vi "PhotonTrackedTarget_Newt.vi"(0 "Pitch":dbl, 1 "Yaw":dbl, 5 "Area":dbl, 7 "Skew":dbl, 9 "FiducalId":i32, 11 "CameraToTarget":T2={"TRANSLATION"={"X"=0.0, "Y"=0.0}, "ROTATION"={"VALUE"=0.0, "COS"=1.0, "SIN"=0.0}, "xF"=FALSE} {"ROTATION"."SIN" format="%13.4f"; "ROTATION"."COS" format="%13.4f"; "ROTATION"."VALUE" format="%13.4f"; "TRANSLATION"."Y" format="%14.3f"; "TRANSLATION"."X" format="%14.3f"}, 13 "TargetCorners":T1[](array[typedef])) -> (4 "TrackedTarget":T5={"Yaw"=0.0, "Pitch"=0.0, "Area"=0.0, "Skew"=0.0, "TargetCorners"=[], "CameraToTarget"={"TRANSLATION"={"X"=0.0, "Y"=0.0}, "ROTATION"={"VALUE"=0.0, "COS"=1.0, "SIN"=0.0}, "xF"=FALSE}, "FiducialId"=0} {"CameraToTarget"."ROTATION"."SIN" format="%13.4f"; "CameraToTarget"."ROTATION"."COS" format="%13.4f"; "CameraToTarget"."ROTATION"."VALUE" format="%13.4f"; "CameraToTarget"."TRANSLATION"."Y" format="%14.3f"; "CameraToTarget"."TRANSLATION"."X" format="%14.3f"})   [LabVIEW 2020, in "PhotonVisionLib.lvlib"]
doc: "Create a new TracedTarget data cluster\n\nInputs:\n - Yaw -- \n - Pitch -- \n - Area -- \n - Skew -- \n - CameraToTarget -- Transform2d\n - TargetCorners -- Array of 4 corners.\n\nOutputs:\n - TrackedTarget -- Created TrackedTarget cluster."
uses:
  PhotonVisionLib.lvlib
  TypeDef/PhotonTrackedTargetType.ctl
  TypeDef/TargetCornerType.ctl
  <vilib>/Rock Robotics/WPI/ThirdParty/JAS_Junk/TrajLib/TypeDef/TRANSFORM2D.ctl
  <vilib>/Rock Robotics/WPI/ThirdParty/JAS_Junk/TrajLib/TypeDef/TRANSLATION2D.ctl
  <vilib>/Rock Robotics/WPI/ThirdParty/JAS_Junk/TrajLib/TypeDef/ROTATION2D.ctl
  <vilib>/Rock Robotics/WPI/ThirdParty/JAS_Junk/TrajLib/Trajectory_Library.lvlib
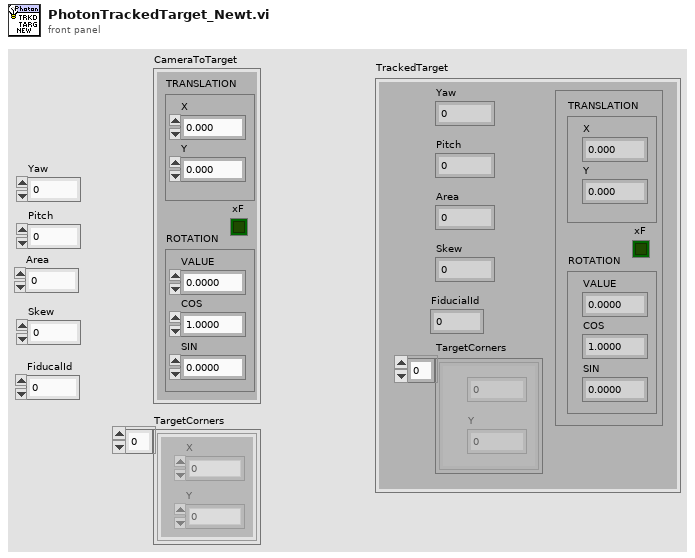
[diagram p1: front panel]
types:
  T1 = typedef "PhotonVisionLib.lvlib/TargetCornerType.ctl" = cluster{"X":dbl, "Y":dbl}
  T2 = typedef "Trajectory_Library.lvlib/TRANSFORM2D.ctl" = cluster{"TRANSLATION":T3, "ROTATION":T4, "xF":bool}
  T3 = typedef "Trajectory_Library.lvlib/TRANSLATION2D.ctl" = cluster{"X":dbl, "Y":dbl}
  T4 = typedef "Trajectory_Library.lvlib/ROTATION2D.ctl" = cluster{"VALUE":dbl, "COS":dbl, "SIN":dbl}
  T5 = typedef "PhotonVisionLib.lvlib/PhotonTrackedTargetType.ctl" = cluster{"Yaw":dbl, "Pitch":dbl, "Area":dbl, "Skew":dbl, "TargetCorners":T1[], "CameraToTarget":T2, "FiducialId":i32}
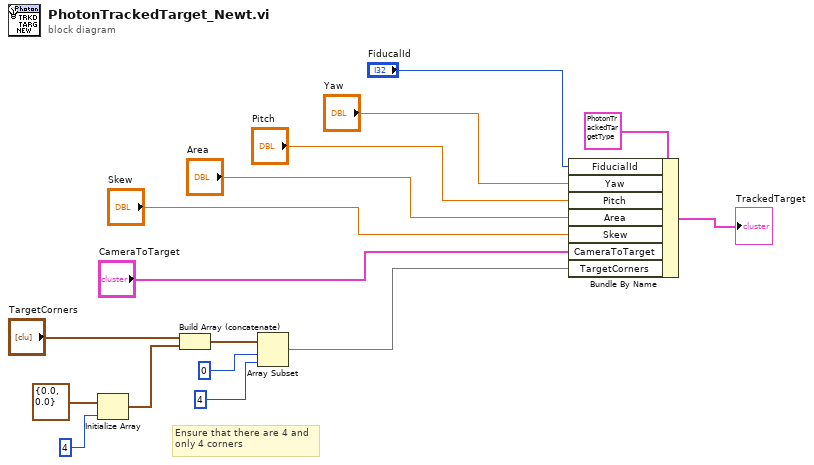
[diagram p0: block diagram]
diagram:
  # "Ensure that there are 4 and \nonly 4 corners"
  n1 = Initialize Array(T1 {"X"=0.0, "Y"=0.0} ("TargetCorner"), 4 ("dimension size")) -> (w6:T1[])
  n2 = Build Array (concatenate)("TargetCorners", w6) -> (w5:T1[])
  n3 = Array Subset(array=w5, index=0, length=4) -> (w2:T1[])
  n4 = Bundle By Name(cluster=T5 {"Yaw"=0.0, "Pitch"=0.0, "Area"=0.0, "Skew"=0.0, "TargetCorners"=[], "CameraToTarget"={"TRANSLATION"={"X"=0.0, "Y"=0.0}, "ROTATION"={"VALUE"=0.0, "COS"=1.0, "SIN"=0.0}, "xF"=FALSE}, "FiducialId"=0} ("PhotonTrackedTarget"), "FiducialId"="FiducalId", "Yaw"="Yaw", "Pitch"="Pitch", "Area"="Area", "Skew"="Skew", "CameraToTarget"="CameraToTarget", "TargetCorners"=w2) -> (→"TrackedTarget":T5)
